vi "DB Insert.vi"(6 "Schema Name":string, 7 "Data":string[][](array[string]), 8 "error in (no error)":errorcluster, 9 "columns":string[](array[string]), 10 "table":string, 11 "Database in":refnum<class "SQLite Database.lvclass">) -> (0 "error out":errorcluster, 2 "SQL":string caption="SQL+ (Col[]) VALUES (?[])", 3 "Database out":refnum<class "SQLite Database.lvclass">)   [LabVIEW 2023, in "HardwareAbstractionLayer_LVOOP.lvlib" / "SQLite Database.lvclass"]
doc: "This VI is DB SQL Insert Query"
uses:
  SQLite Database.lvclass
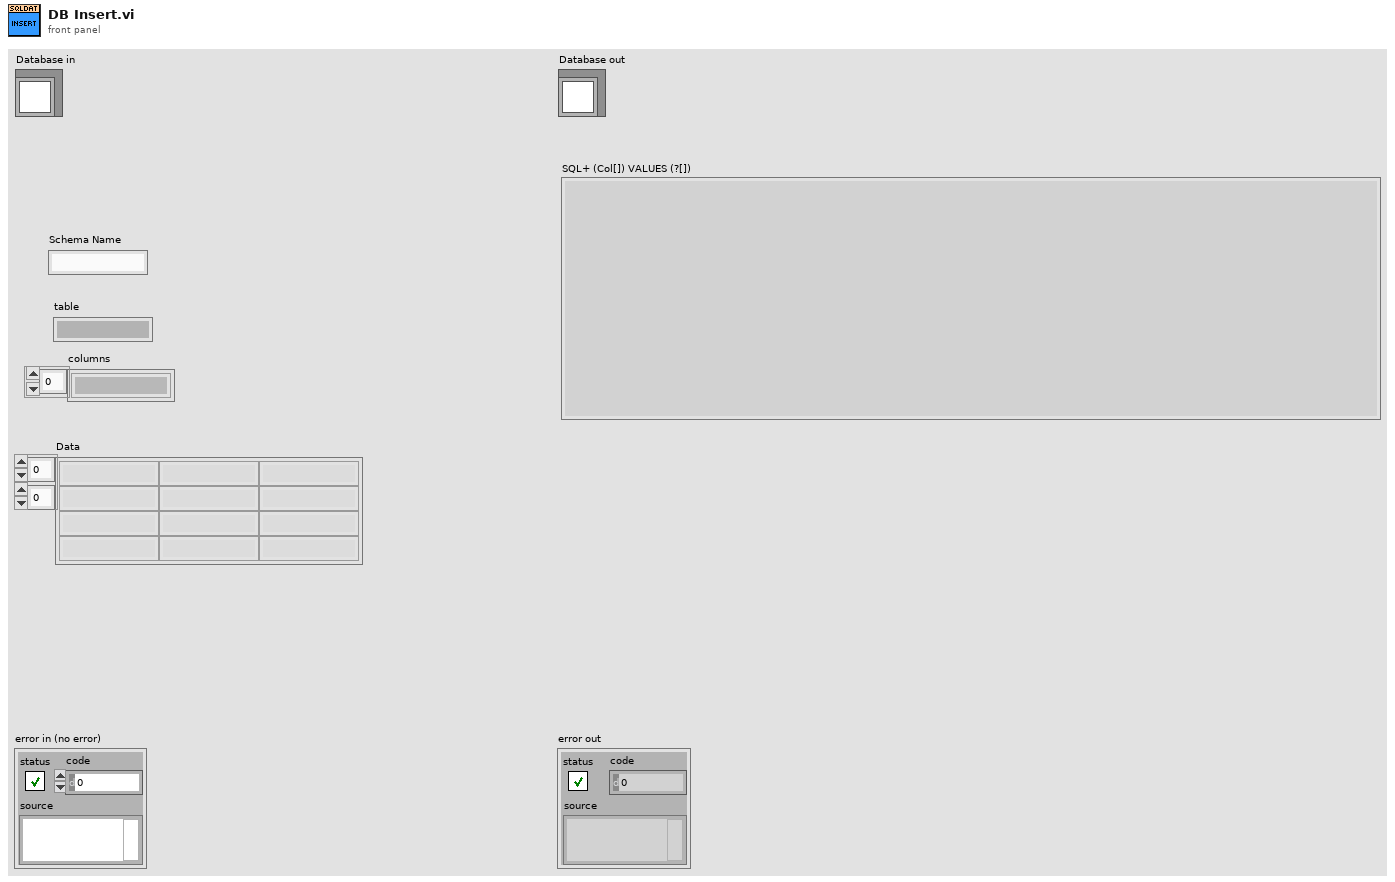
[diagram p1: front panel]
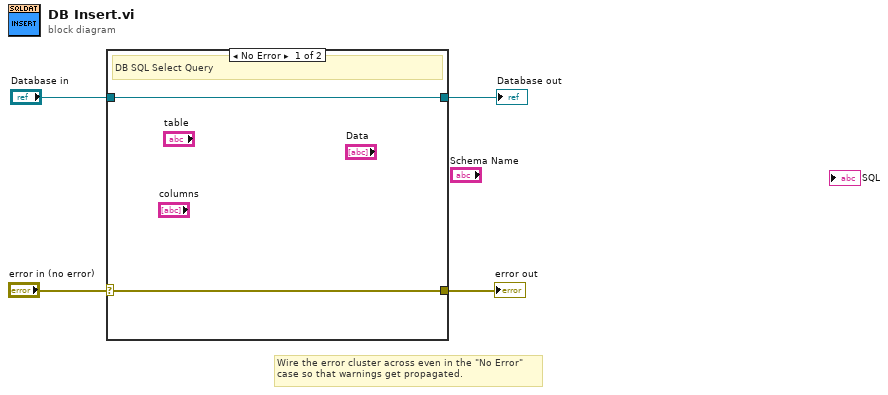
[diagram p0: block diagram]
diagram:
  # "Wire the error cluster across even in the \"No Error\"\ncase so that warnings get propagated."
  n1 = case shown="No Error" "error in (no error)" {
    selector: "error in (no error)" -> [w5 w8]
    tunnel: [w5 w8] -> w3
    tunnel: [w6 w7] -> w1
    tunnel: "Database in" -> [w6 w7]
    frame No Error {
      # "DB SQL Select Query"
    }
    frame Error {
    }
  }
  "error out" <- w3
  "Database out" <- w1
